vi "Exit.vi"(8 "error in (no error)":errorcluster, 11 "Object ref in":T1) -> (0 "error out":errorcluster, 3 "Object ref out":T1)   [LabVIEW 2013, in "HardwareCharacterization.lvlib" / "HC-Main.lvclass"]
uses:
  HC-Main.lvclass
  Object-reference.ctl
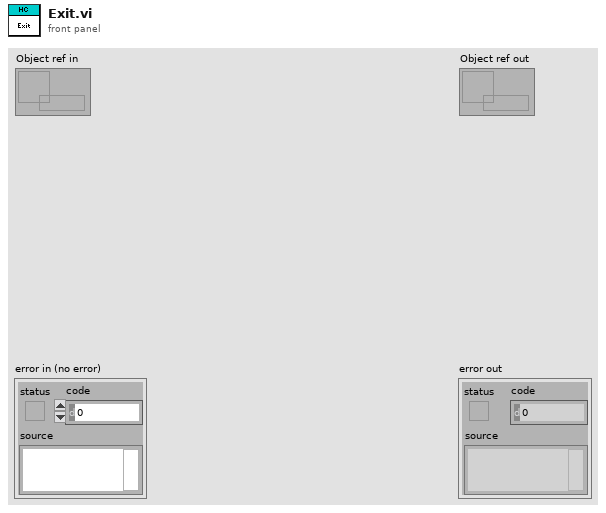
[diagram p1: front panel]
types:
  T1 = typedef "HardwareCharacterization.lvlib/HC-Main.lvclass/Object-reference.ctl" = refnum<data-value>
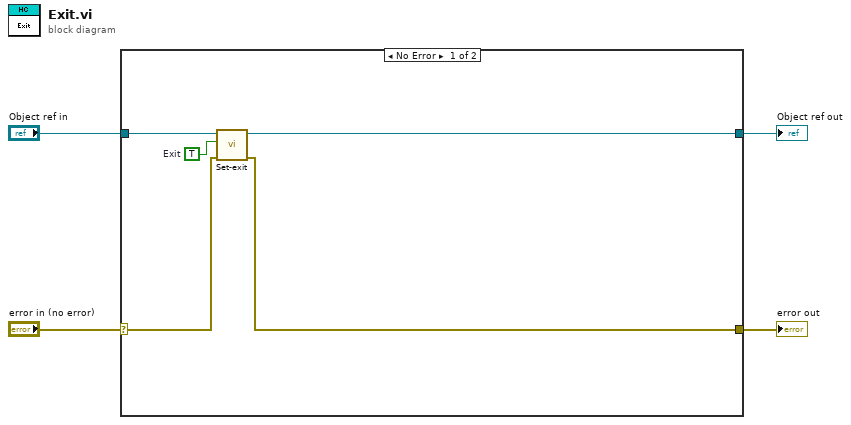
[diagram p0: block diagram]
diagram:
  n1 = case shown="No Error" "error in (no error)" {
    selector: "error in (no error)" -> [w7 w11]
    tunnel: [w5 w11] -> w3
    tunnel: [w6 w10] -> w1
    tunnel: "Object ref in" -> [w8 w10]
    frame No Error {
      w9 = TRUE  # Exit
      n2 = call "Set-exit.vi"("error in (no error)"=w7, "Exit?"=w9, "Object ref in"=w8) -> ("error out"=w5:errorcluster, "Object ref out"=w6:T1)  [unwired: 7 in]
    }
    frame Error {
    }
  }
  "error out" <- w3
  "Object ref out" <- w1
